vi "电缸控制.vi"(1 "步序号":u32, 2 "枚举":enum16{"开机", "返回原点", "定位运转", "报警复位"}(ring), 3 "输出设备":tag) -> (0 "error out":errorcluster caption="错误输出")   [LabVIEW 2014]
uses:
  <vilib>/DAQmx/create/channels.llb/DAQmx Create Channel (DO-Digital Output).vi
  <vilib>/DAQmx/write.llb/DAQmx Write (Digital 1D Bool 1Chan 1Samp).vi
panel:
  in  "步信息":T1
  in  "人工输出":T2
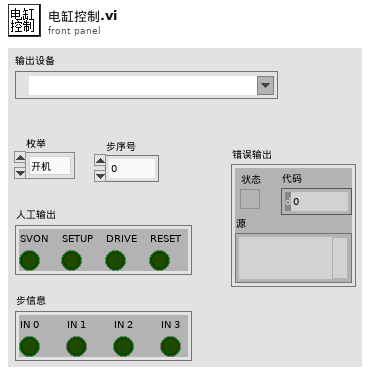
[diagram p1: front panel]
types:
  T1 = cluster{"IN 0":bool, "IN 1":bool, "IN 2":bool, "IN 3":bool}
  T2 = cluster{"SVON":bool, "SETUP":bool, "DRIVE":bool, "RESET":bool}
  T3 = cluster{"Boolean array[0]":bool, "Boolean array[1]":bool, "Boolean array[2]":bool, "Boolean array[3]":bool}
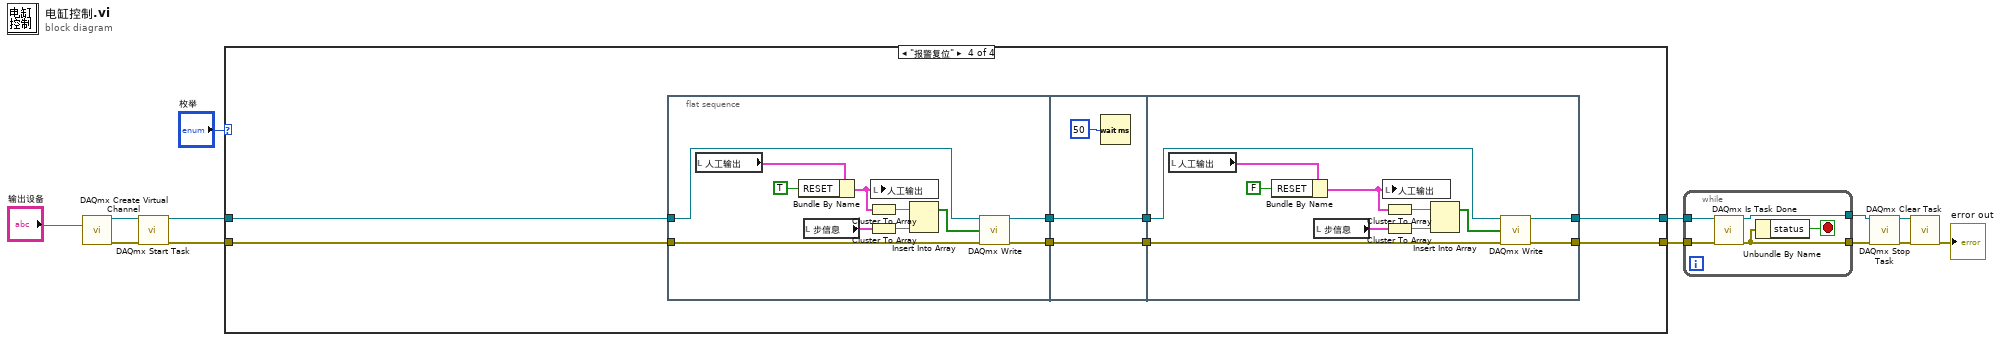
[diagram p0: block diagram]
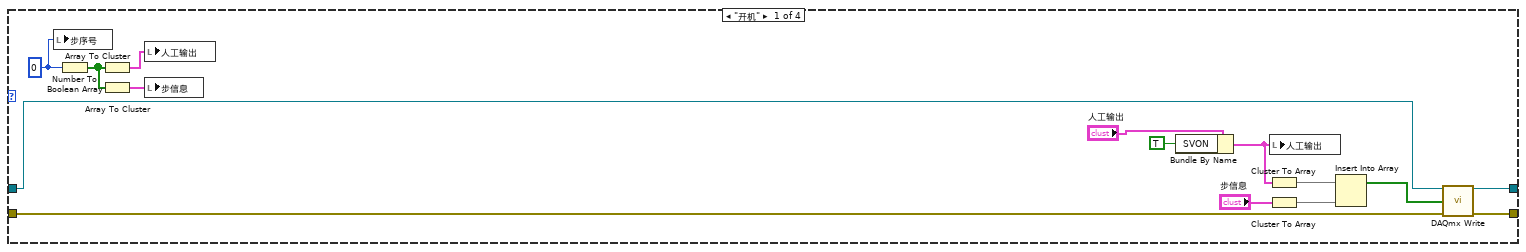
[diagram p2: hidden frame]
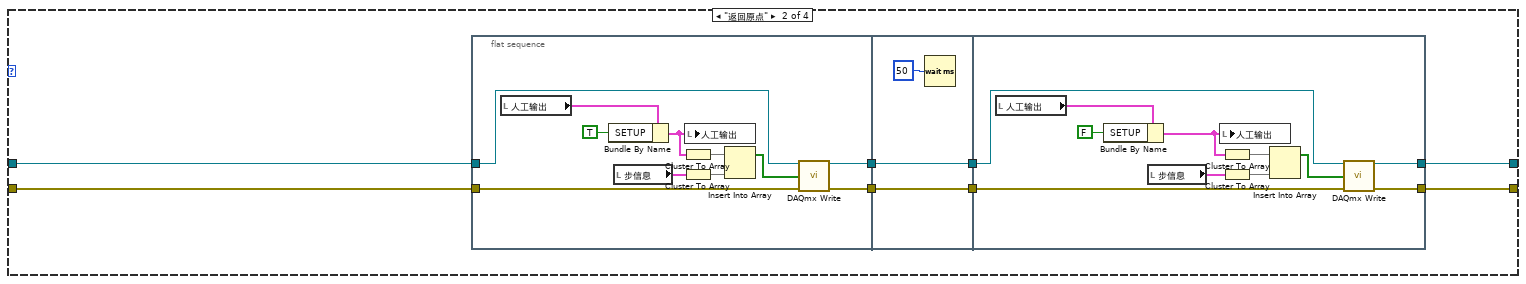
[diagram p3: hidden frame]
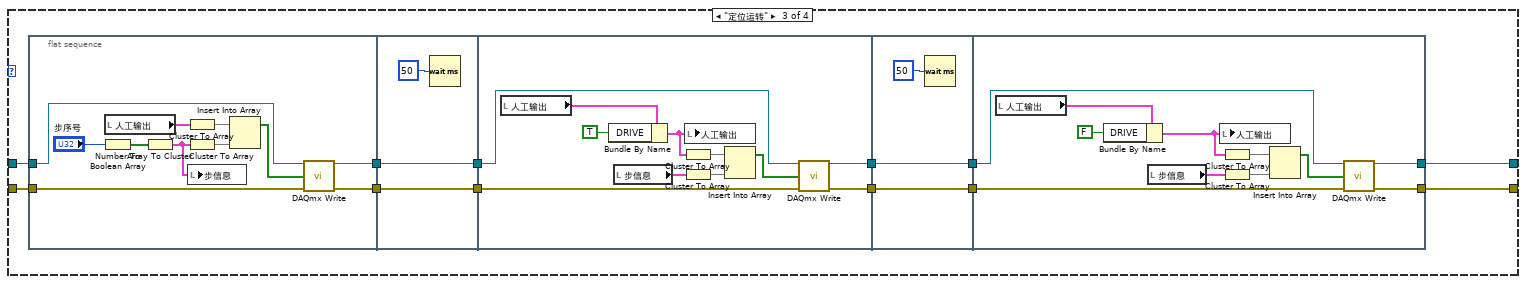
[diagram p4: hidden frame]
diagram:
  n1 = call-poly <vilib>:"DAQmx Create Virtual Channel.vi"("lines"="输出设备") -> ("task out"=w11:refnum<k21>, "error out"=w12:errorcluster)  [unwired: 13 in]
  n2 = call <vilib>:"DAQmx Start Task.vi"("task/channels in"=w11, "error in"=w12) -> ("task out"=w9:refnum<k21>, "error out"=w8:errorcluster)  [unwired: 12 in]
  n3 = case shown="\"报警复位\"" "枚举" {
    tunnel: w9 -> [w25 w36 w73 w120]
    tunnel: w8 -> [w24 w35 w72 w119]
    tunnel: [w22 w34 w67 w114] -> w3
    tunnel: [w21 w33 w66 w113] -> w2
    frame "开机" {
      w17 = 0
      n4 = local write "步序号"(w17) -> ()
      n5 = Number To Boolean Array(number=w17) -> (Boolean array=w16:bool[])
      n6 = Array To Cluster(array=w16) -> (cluster=w15:T3)
      n7 = Array To Cluster(array=w16) -> (cluster=w14:T3)
      n8 = local write "人工输出"(w15) -> ()
      n9 = local write "步信息"(w14) -> ()
      n10 = Bundle By Name(cluster="人工输出", "SVON"=TRUE) -> (w18:T2)
      n11 = Cluster To Array(cluster=w18) -> (array=w27:bool[])
      n12 = Cluster To Array(cluster="步信息") -> (array=w26:bool[])
      n13 = local write "人工输出"(w18) -> ()
      n14 = Insert Into Array(array=w27, new element=w26) -> (w23:bool[])  [unwired: 1 in]
      n15 = call-poly <vilib>:"DAQmx Write.vi"("task/channels in"=w25, "data"=w23, "error in"=w24) -> ("task out"=w22:refnum<k21>, "error out"=w21:errorcluster)  [unwired: 10 in, 1 out]
    }
    frame "返回原点" {
      n16 = flat-sequence {
        tunnel: w36 -> [w47]
        tunnel: w35 -> [w46]
        tunnel: [w39] -> w32
        tunnel: [w38] -> w30
        tunnel: w32 -> [w49]
        tunnel: [w49] -> w31
        tunnel: w30 -> [w48]
        tunnel: [w48] -> w29
        tunnel: [w61] -> w34
        tunnel: [w60] -> w33
        tunnel: w31 -> [w52]
        tunnel: w29 -> [w51]
        frame #0 {
          n17 = local read "人工输出"() -> (w45:T2)
          n18 = Bundle By Name(cluster=w45, "SETUP"=TRUE) -> (w43:T2)
          n19 = local read "步信息"() -> (w41:T1)
          n20 = Cluster To Array(cluster=w43) -> (array=w42:bool[])
          n21 = Cluster To Array(cluster=w41) -> (array=w37:bool[])
          n22 = local write "人工输出"(w43) -> ()
          n23 = Insert Into Array(array=w42, new element=w37) -> (w40:bool[])  [unwired: 1 in]
          n24 = call-poly <vilib>:"DAQmx Write.vi"("task/channels in"=w47, "data"=w40, "error in"=w46) -> ("task out"=w39:refnum<k21>, "error out"=w38:errorcluster)  [unwired: 10 in, 1 out]
        }
        frame #1 {
          n25 = Wait (ms)(milliseconds to wait=u32 50 ("等待时间（毫秒）")) -> ()  [unwired: 1 out]
        }
        frame #2 {
          n26 = local read "人工输出"() -> (w59:T2)
          n27 = Bundle By Name(cluster=w59, "SETUP"=FALSE) -> (w57:T2)
          n28 = local read "步信息"() -> (w56:T1)
          n29 = local write "人工输出"(w57) -> ()
          n30 = Cluster To Array(cluster=w57) -> (array=w55:bool[])
          n31 = Cluster To Array(cluster=w56) -> (array=w54:bool[])
          n32 = Insert Into Array(array=w55, new element=w54) -> (w53:bool[])  [unwired: 1 in]
          n33 = call-poly <vilib>:"DAQmx Write.vi"("task/channels in"=w52, "data"=w53, "error in"=w51) -> ("task out"=w61:refnum<k21>, "error out"=w60:errorcluster)  [unwired: 10 in, 1 out]
        }
      }
    }
    frame "定位运转" {
      n34 = flat-sequence {
        tunnel: w73 -> [w79]
        tunnel: w72 -> [w78]
        tunnel: [w75] -> w71
        tunnel: [w74] -> w68
        tunnel: w71 -> [w86]
        tunnel: [w86] -> w70
        tunnel: [w85] -> w69
        tunnel: w68 -> [w85]
        tunnel: w70 -> [w98]
        tunnel: w69 -> [w97]
        tunnel: [w89] -> w65
        tunnel: [w88] -> w62
        tunnel: w65 -> [w100]
        tunnel: [w100] -> w64
        tunnel: [w99] -> w63
        tunnel: w62 -> [w99]
        tunnel: [w110] -> w67
        tunnel: [w109] -> w66
        tunnel: w64 -> [w108]
        tunnel: w63 -> [w107]
        frame #0 {
          n35 = Number To Boolean Array(number="步序号") -> (Boolean array=w83:bool[])
          n36 = local read "人工输出"() -> (w81:T2)
          n37 = Array To Cluster(array=w83) -> (cluster=w76:T3)
          n38 = Cluster To Array(cluster=w81) -> (array=w80:bool[])
          n39 = Cluster To Array(cluster=w76) -> (array=w82:bool[])
          n40 = local write "步信息"(w76) -> ()
          n41 = Insert Into Array(array=w80, new element=w82) -> (w77:bool[])  [unwired: 1 in]
          n42 = call-poly <vilib>:"DAQmx Write.vi"("task/channels in"=w79, "data"=w77, "error in"=w78) -> ("task out"=w75:refnum<k21>, "error out"=w74:errorcluster)  [unwired: 10 in, 1 out]
        }
        frame #1 {
          n43 = Wait (ms)(milliseconds to wait=u32 50 ("毫秒倍数")) -> ()  [unwired: 1 out]
        }
        frame #2 {
          n44 = local read "人工输出"() -> (w96:T2)
          n45 = Bundle By Name(cluster=w96, "DRIVE"=TRUE) -> (w94:T2)
          n46 = local read "步信息"() -> (w93:T1)
          n47 = Cluster To Array(cluster=w94) -> (array=w92:bool[])
          n48 = Cluster To Array(cluster=w93) -> (array=w91:bool[])
          n49 = local write "人工输出"(w94) -> ()
          n50 = Insert Into Array(array=w92, new element=w91) -> (w90:bool[])  [unwired: 1 in]
          n51 = call-poly <vilib>:"DAQmx Write.vi"("task/channels in"=w98, "data"=w90, "error in"=w97) -> ("task out"=w89:refnum<k21>, "error out"=w88:errorcluster)  [unwired: 10 in, 1 out]
        }
        frame #3 {
          n52 = Wait (ms)(milliseconds to wait=u32 50 ("毫秒倍数")) -> ()  [unwired: 1 out]
        }
        frame #4 {
          n53 = local read "人工输出"() -> (w112:T2)
          n54 = Bundle By Name(cluster=w112, "DRIVE"=FALSE) -> (w106:T2)
          n55 = local read "步信息"() -> (w105:T1)
          n56 = local write "人工输出"(w106) -> ()
          n57 = Cluster To Array(cluster=w106) -> (array=w104:bool[])
          n58 = Cluster To Array(cluster=w105) -> (array=w103:bool[])
          n59 = Insert Into Array(array=w104, new element=w103) -> (w102:bool[])  [unwired: 1 in]
          n60 = call-poly <vilib>:"DAQmx Write.vi"("task/channels in"=w108, "data"=w102, "error in"=w107) -> ("task out"=w110:refnum<k21>, "error out"=w109:errorcluster)  [unwired: 10 in, 1 out]
        }
      }
    }
    frame "报警复位" {
      n61 = flat-sequence {
        tunnel: w120 -> [w131]
        tunnel: w119 -> [w130]
        tunnel: [w122] -> w118
        tunnel: [w121] -> w115
        tunnel: w118 -> [w133]
        tunnel: [w133] -> w117
        tunnel: [w132] -> w116
        tunnel: w115 -> [w132]
        tunnel: w117 -> [w139]
        tunnel: w116 -> [w138]
        tunnel: [w136] -> w114
        tunnel: [w135] -> w113
        frame #0 {
          n62 = local read "人工输出"() -> (w129:T2)
          n63 = Bundle By Name(cluster=w129, "RESET"=TRUE) -> (w127:T2)
          n64 = local read "步信息"() -> (w126:T1)
          n65 = Cluster To Array(cluster=w127) -> (array=w125:bool[])
          n66 = Cluster To Array(cluster=w126) -> (array=w124:bool[])
          n67 = local write "人工输出"(w127) -> ()
          n68 = Insert Into Array(array=w125, new element=w124) -> (w123:bool[])  [unwired: 1 in]
          n69 = call-poly <vilib>:"DAQmx Write.vi"("task/channels in"=w131, "data"=w123, "error in"=w130) -> ("task out"=w122:refnum<k21>, "error out"=w121:errorcluster)  [unwired: 10 in, 1 out]
        }
        frame #1 {
          n70 = Wait (ms)(milliseconds to wait=u32 50 ("毫秒倍数")) -> ()  [unwired: 1 out]
        }
        frame #2 {
          n71 = local read "人工输出"() -> (w144:T2)
          n72 = Bundle By Name(cluster=w144, "RESET"=FALSE) -> (w140:T2)
          n73 = local read "步信息"() -> (w141:T1)
          n74 = local write "人工输出"(w140) -> ()
          n75 = Cluster To Array(cluster=w140) -> (array=w143:bool[])
          n76 = Cluster To Array(cluster=w141) -> (array=w142:bool[])
          n77 = Insert Into Array(array=w143, new element=w142) -> (w137:bool[])  [unwired: 1 in]
          n78 = call-poly <vilib>:"DAQmx Write.vi"("task/channels in"=w139, "data"=w137, "error in"=w138) -> ("task out"=w136:refnum<k21>, "error out"=w135:errorcluster)  [unwired: 10 in, 1 out]
        }
      }
    }
  }
  n79 = while {
    tunnel: [w150] -> w7
    tunnel: [w149] -> w6
    tunnel: w3 -> [w147]
    tunnel: w2 -> [w146]
    stop <- w148 stop-if-true
    n80 = call <vilib>:"DAQmx Is Task Done.vi"("task/channels in"=w147, "error in"=w146) -> ("task out"=w150:refnum<k21>, "error out"=w149:errorcluster)  [unwired: 11 in, 1 out]
    n81 = Unbundle By Name(w149) -> ("status"=w148:bool)
  }
  n82 = call <vilib>:"DAQmx Stop Task.vi"("task/channels in"=w7, "error in"=w6) -> ("task out"=w5:refnum<k21>, "error out"=w4:errorcluster)  [unwired: 12 in]
  n83 = call <vilib>:"DAQmx Clear Task.vi"("task in"=w5, "error in"=w4) -> ("error out"=→"error out":errorcluster)  [unwired: 13 in]
